vi "Global.vi"() -> ()   [LabVIEW 2011, in "PXIe-433x Custom Device.lvlib"]
uses:
  PXIe-433x Custom Device.lvlib
panel:
  in  "DrvRTSI0?":string="DrvRTSI0?"
  in  "Mode":string="Mode"
  in  "HW Rate":string="HW Rate"
  in  "Core Assignment":string="Core Assignment"
  in  "Master type":string="Master type"
  in  "Main Enabled":string="FE85F79D-11A6-F784-7D58-7AF897158418"
  in  "Main Disabled":string="BC1EFC41-E47A-AED7-5F6C-233661952A37"
  in  "Card Page GUID":string="08B33A5F-7DFA-3EF9-05C6-5710A7STCARD"
  in  "Scale Type":string="Scaling Type"
  in  "Scaling Info":string="Scaling Info"
  in  "Sensor Type":string="Sensor Type"
  in  "DeviceName":string="DeviceName"
  in  "Bridge Info":string="Bridge Info"
  in  "Min Val":string="Min Val"
  in  "Max Val":string="Max Val"
  in  "Channel Page GUID":string="08B33A5F-7DFA-3EF9-05C6-5710A7STRAIN"
  in  "Channel #":string="Channel #"
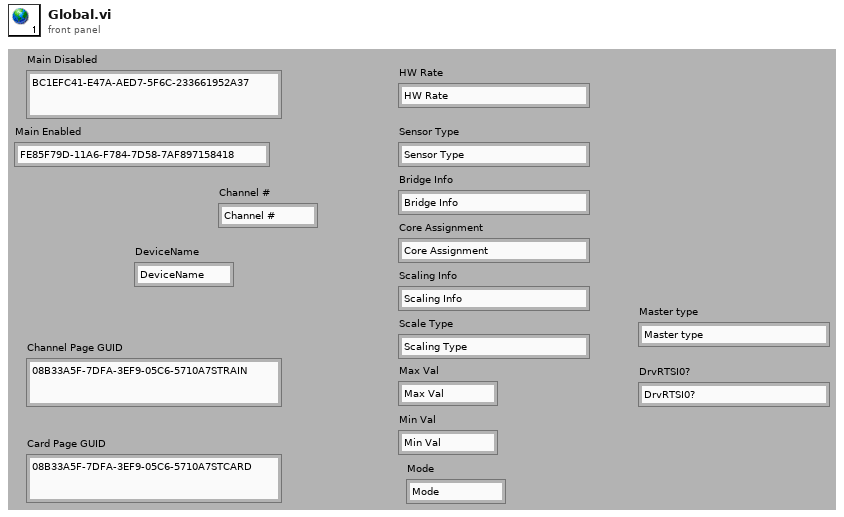
[diagram p1: front panel]
diagram:
